vi "acel_processing.vi"(7 "rate":dbl, 8 "error in":errorcluster, 11 "acelData":dbl[][](array[numeric])) -> (0 "error out":errorcluster, 3 "RMS":dbl[](array[numeric]))   [LabVIEW 2016]
uses:
  MainFGV/MainFGV_mods.ctl
  <vilib>/Analysis/5stat.llb/RMS (DBL).vi
  <vilib>/Analysis/NI_AALPro.lvlib
panel:
  out "size(s)":i32[](array[numeric])
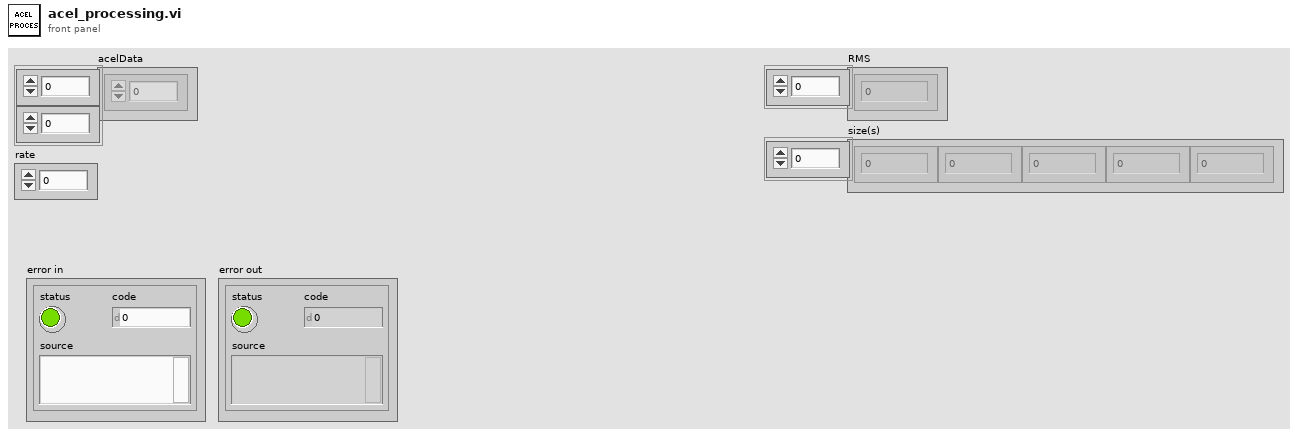
[diagram p1: front panel]
types:
  T1 = typedef "MainFGV_mods.ctl" = enum16{"Init", "Config", "CreateTask", "Register", "Acquire", "Start", "Burst", "Record", "End"}
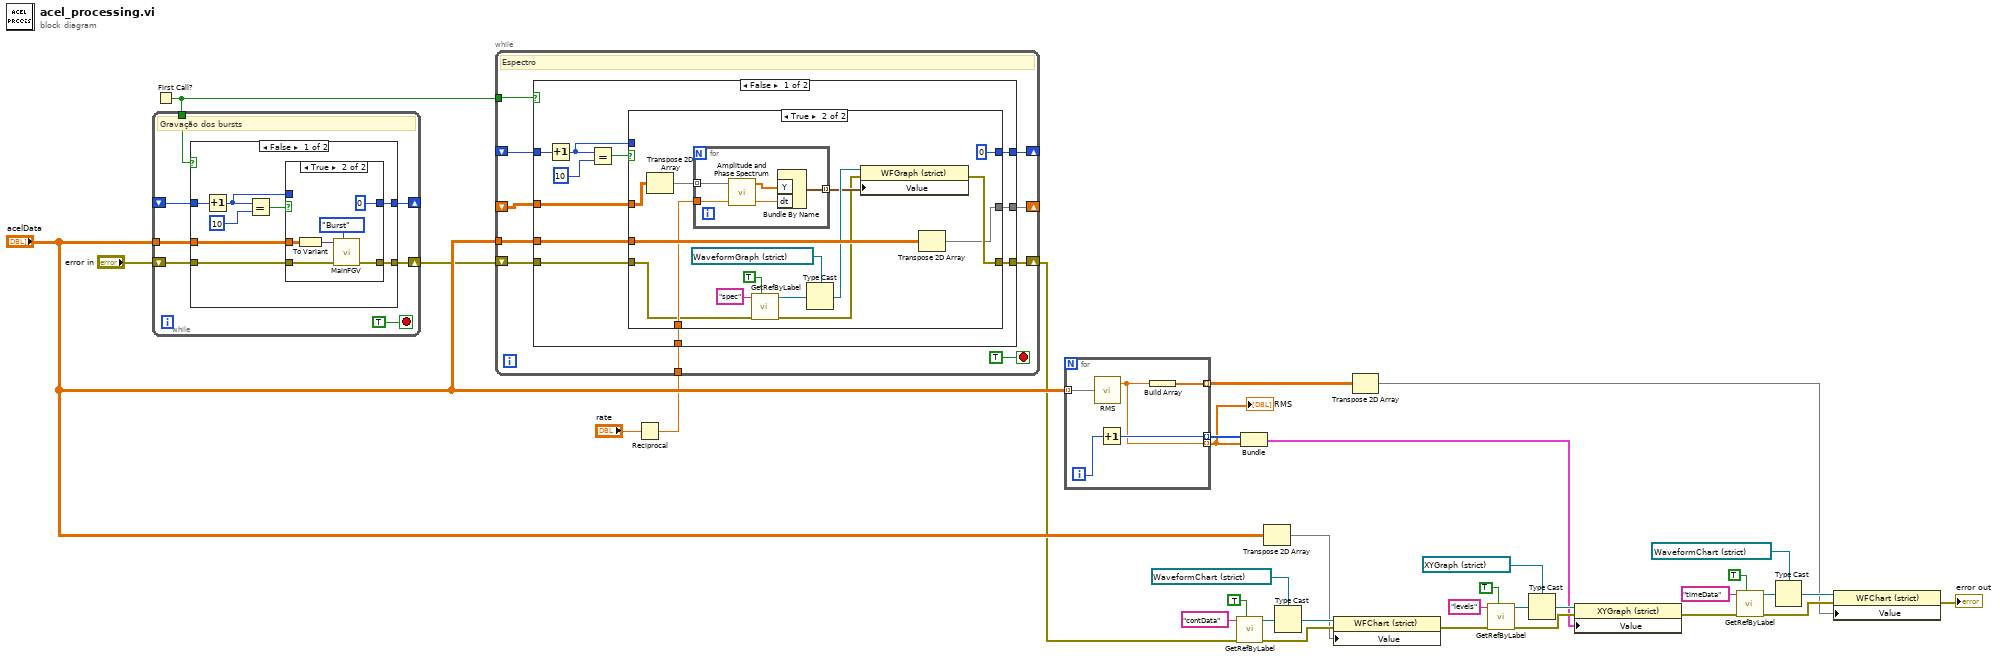
[diagram p0: block diagram]
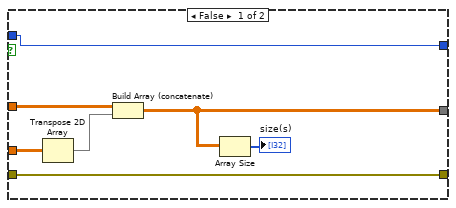
[diagram p2: hidden frame]
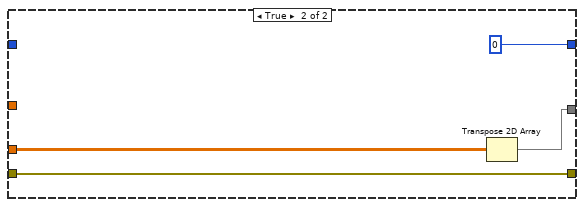
[diagram p3: hidden frame]
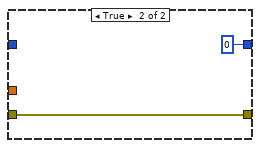
[diagram p5: hidden frame]
diagram:
  n1 = First Call?() -> (First Call?: T/F=w4:bool)
  n2 = while {
    shift-right: [w40] -> _
    shift-left: _ -> [w39]
    shift-right: [w36] -> w5
    shift-left: "error in" -> [w38]
    tunnel: "acelData" -> [w37]
    tunnel: w4 -> [w35]
    stop <- TRUE stop-if-true
    # "Gravação dos bursts"
    n3 = case shown="False" w35 {
      tunnel: [w46 0] -> w40
      tunnel: w39 -> [w49 _]
      tunnel: w38 -> [w45 w58]
      tunnel: w37 -> [w44 _]
      tunnel: [w43 w58] -> w36
      frame False {
        n4 = Increment(x=w49) -> (x+1=w42:i32)
        n5 = Equal?(x=w42, y=10) -> (x = y?=w47:bool)
        n6 = case shown="True" w47 {
          tunnel: [w51 0 ("y")] -> w46
          tunnel: w45 -> [w50 w54]
          tunnel: w44 -> [_ w53]
          tunnel: [w50 w52] -> w43
          tunnel: w42 -> [w51 _]
          frame False {
          }
          frame True {
            n7 = To Variant(anything=w53) -> (Variant=w56:variant)
            n8 = call "MainFGV.vi"("FGV_mods"=MainFGV_mods."Burst", "Error In"=w54, "DataIn"=w56) -> ("Error Out"=w52:errorcluster)  [unwired: 7 in, 1 out]
          }
        }
      }
      frame True {
      }
    }
  }
  n9 = Reciprocal(x="rate") -> (1/x=w3:dbl)
  n10 = while {
    shift-right: [w68] -> _
    shift-left: _ -> [w67]
    shift-right: [w64] -> w2
    shift-left: w5 -> [w66]
    tunnel: "acelData" -> [w65]
    tunnel: w4 -> [w63]
    shift-right: [w62] -> _
    shift-left: _ -> [w61]
    tunnel: w3 -> [w60]
    stop <- TRUE stop-if-true
    # "Espectro"
    n11 = case shown="False" w63 {
      tunnel: [w77 0] -> w68
      tunnel: w67 -> [w80 _]
      tunnel: w66 -> [w76 w110]
      tunnel: w65 -> [w75 w109]
      tunnel: [w74 w110] -> w64
      tunnel: [w72 w108] -> w62
      tunnel: w61 -> [w71 _]
      tunnel: w60 -> [w70 _]
      frame False {
        n12 = Increment(x=w80) -> (x+1=w73:i32)
        n13 = Equal?(x=w73, y=10) -> (x = y?=w78:bool)
        n14 = case shown="True" w78 {
          tunnel: [w87 0 ("y")] -> w77
          tunnel: w76 -> [w86 w96]
          tunnel: w75 -> [w83 w101]
          tunnel: [w86 w90] -> w74
          tunnel: w73 -> [w87 _]
          tunnel: [w81 w88] -> w72
          tunnel: w71 -> [w85 w100]
          tunnel: w70 -> [_ w99]
          frame False {
            n15 = Transpose 2D Array(2D array=w83) -> (transposed array=w82:dbl[][])
            n16 = Build Array (concatenate)(w85, w82) -> (w81:dbl[][])
            n17 = Array Size(array=w81) -> (size(s)=→"size(s)":i32[])
          }
          frame True {
            n18 = Transpose 2D Array(2D array=w100) -> (transposed array=w89:dbl[][])
            n19 = for {
              tunnel: w89 -> [w105] mode=indexing
              tunnel: w99 -> [w104]
              tunnel: [w103] -> w92 mode=indexing
              n20 = call <vilib>:"Amplitude and Phase Spectrum.vi"("dt"=w104, "Signal (V)"=w105) -> ("df"=w107:dbl, "Amp Spectrum Mag (Vrms)"=w106:dbl[])  [unwired: 1 in, 1 out]
              n21 = Bundle By Name("Y"=w106, "dt"=w107) -> (w103:waveform(dbl))  [unwired: 1 in]
            }
            n22 = call "GetRefByLabel.vi"("InsideTab"=TRUE, "error in"=w96, "Label"="spec") -> ("error out"=w91:errorcluster, "Ctl Refnum"=w97:refnum<vi>)  [unwired: 6 in, 1 out]
            n23 = Type Cast(type=refnum<vi> refnum ("spec"), x=w97) -> (*(type *) &x=w93:refnum<vi>)
            n24 = property class="WFGraph (strict)"(reference=w93, error in=w91, "Value"=w92) -> (error out=w90:errorcluster)  [unwired: 1 out]
            n25 = Transpose 2D Array(2D array=w101) -> (transposed array=w88:dbl[][])
          }
        }
      }
      frame True {
        n26 = Transpose 2D Array(2D array=w109) -> (transposed array=w108:dbl[][])
      }
    }
  }
  n27 = for {
    tunnel: "acelData" -> [w112] mode=indexing
    tunnel: [w115] -> w20 mode=indexing
    tunnel: [w114] -> w34 mode=indexing
    tunnel: [w113] -> w9 mode=indexing
    i -> [w116]
    n28 = call-poly <vilib>:"RMS.vi"("X"=w112) -> ("rms value"=w113:dbl)  [unwired: 1 out]
    n29 = Increment(x=w116) -> (x+1=w114:i32)
    n30 = Build Array(w113) -> (w115:dbl[])
  }
  "RMS" <- w9
  n31 = call "GetRefByLabel.vi"("InsideTab"=TRUE, "error in"=w2, "Label"="contData") -> ("error out"=w14:errorcluster, "Ctl Refnum"=w15:refnum<vi>)  [unwired: 6 in, 1 out]
  n32 = Bundle(w34, w9) -> (w28:cluster{i32[], dbl[]})  [unwired: 1 in]
  n33 = Transpose 2D Array(2D array="acelData") -> (transposed array=w10:dbl[][])
  n34 = Type Cast(type=refnum<vi> refnum ("timeData"), x=w15) -> (*(type *) &x=w16:refnum<vi>)
  n35 = property class="WFChart (strict)"(reference=w16, error in=w14, "Value"=w10) -> (error out=w11:errorcluster)  [unwired: 1 out]
  n36 = Transpose 2D Array(2D array=w20) -> (transposed array=w1:dbl[][])
  n37 = call "GetRefByLabel.vi"("InsideTab"=TRUE, "error in"=w11, "Label"="levels") -> ("error out"=w29:errorcluster, "Ctl Refnum"=w31:refnum<vi>)  [unwired: 6 in, 1 out]
  n38 = Type Cast(type=refnum<vi> refnum ("levels"), x=w31) -> (*(type *) &x=w30:refnum<vi>)
  n39 = property class="XYGraph (strict)"(reference=w30, error in=w29, "Value"=w28) -> (error out=w25:errorcluster)  [unwired: 1 out]
  n40 = call "GetRefByLabel.vi"("InsideTab"=TRUE, "error in"=w25, "Label"="timeData") -> ("error out"=w23:errorcluster, "Ctl Refnum"=w22:refnum<vi>)  [unwired: 6 in, 1 out]
  n41 = Type Cast(type=refnum<vi> refnum ("timeData"), x=w22) -> (*(type *) &x=w21:refnum<vi>)
  n42 = property class="WFChart (strict)"(reference=w21, error in=w23, "Value"=w1) -> (error out=→"error out":errorcluster)  [unwired: 1 out]
